vi "报警信息.vi"(11 "报警簇":T1) -> (2 "系统报警信息":string, 3 "采配水报警信息":string)   [LabVIEW 2016, in "PLC.lvlib"]
uses:
  PLC.lvlib
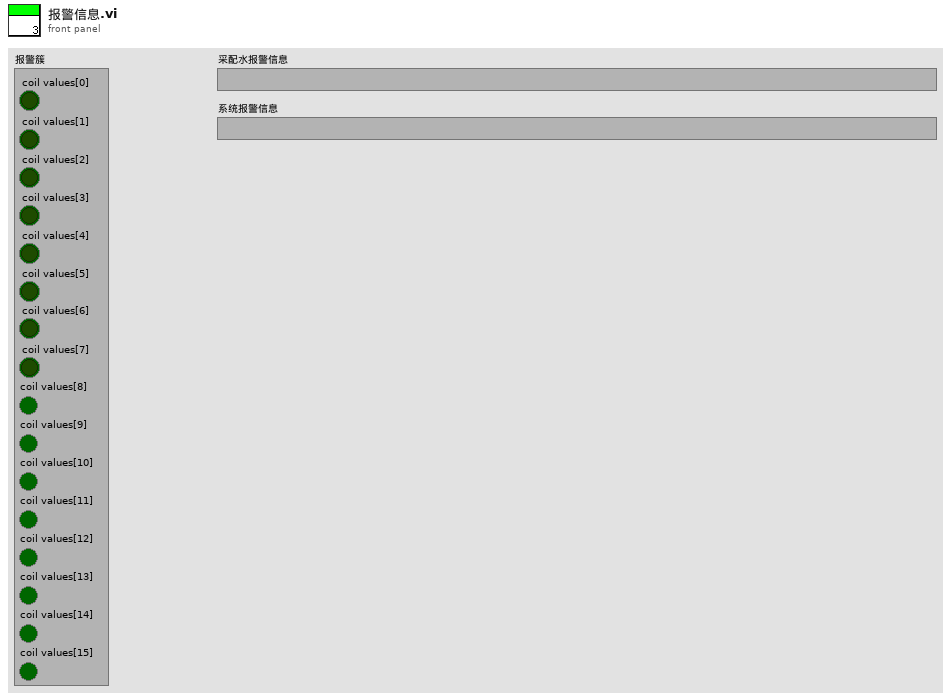
[diagram p1: front panel]
types:
  T1 = cluster{"coil values[0]":bool, "coil values[1]":bool, "coil values[2]":bool, "coil values[3]":bool, "coil values[4]":bool, "coil values[5]":bool, "coil values[6]":bool, "coil values[7]":bool, "coil values[8]":bool, "coil values[9]":bool, "coil values[10]":bool, "coil values[11]":bool, "coil values[12]":bool, "coil values[13]":bool, "coil values[14]":bool, "coil values[15]":bool}
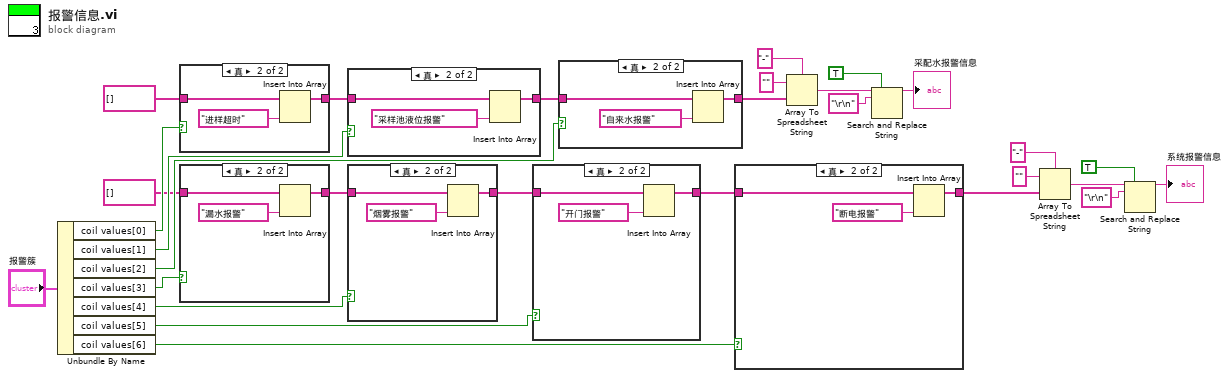
[diagram p0: block diagram]
diagram:
  n1 = Unbundle By Name("报警簇") -> ("coil values[0]"=w28:bool, "coil values[1]"=w27:bool, "coil values[2]"=w22:bool, "coil values[3]"=w21:bool, "coil values[4]"=w20:bool, "coil values[5]"=w19:bool, "coil values[6]"=w18:bool)
  n2 = case shown="真" w28 {
    tunnel: string[] [] -> [w30 w32]
    tunnel: [w30 w31] -> w23
    frame False {
    }
    frame True {
      n3 = Insert Into Array(array=w32, new element="进样超时" ("组合框")) -> (w31:string[])  [unwired: 1 in]
    }
  }
  n4 = case shown="真" w21 {
    tunnel: string[] [] -> [w34 w37]
    tunnel: [w34 w35] -> w17
    frame False {
    }
    frame True {
      n5 = Insert Into Array(array=w37, new element="漏水报警" ("组合框")) -> (w35:string[])  [unwired: 1 in]
    }
  }
  n6 = case shown="真" w27 {
    tunnel: w23 -> [w38 w41]
    tunnel: [w38 w39] -> w10
    frame False {
    }
    frame True {
      n7 = Insert Into Array(array=w41, new element="采样池液位报警" ("组合框")) -> (w39:string[])  [unwired: 1 in]
    }
  }
  n8 = case shown="真" w20 {
    tunnel: w17 -> [w42 w45]
    tunnel: [w42 w43] -> w16
    frame False {
    }
    frame True {
      n9 = Insert Into Array(array=w45, new element="烟雾报警" ("组合框")) -> (w43:string[])  [unwired: 1 in]
    }
  }
  n10 = case shown="真" w19 {
    tunnel: w16 -> [w46 w49]
    tunnel: [w46 w47] -> w15
    frame False {
    }
    frame True {
      n11 = Insert Into Array(array=w49, new element="开门报警" ("组合框")) -> (w47:string[])  [unwired: 1 in]
    }
  }
  n12 = case shown="真" w22 {
    tunnel: w10 -> [w50 w51]
    tunnel: [w50 w52] -> w9
    frame False {
    }
    frame True {
      n13 = Insert Into Array(array=w51, new element="自来水报警" ("组合框")) -> (w52:string[])  [unwired: 1 in]
    }
  }
  n14 = case shown="真" w18 {
    tunnel: w15 -> [w54 w57]
    tunnel: [w54 w55] -> w14
    frame False {
    }
    frame True {
      n15 = Insert Into Array(array=w57, new element="断电报警" ("组合框")) -> (w55:string[])  [unwired: 1 in]
    }
  }
  n16 = Array To Spreadsheet String(delimiter (Tab)="-" ("分隔符(Tab)"), array=w9, 3:"" ("格式字符串")) -> (spreadsheet string=w2:string)
  n17 = Search and Replace String(replace all?=TRUE ("替换全部？(F)"), input string=w2, search string="\r\n" ("搜索字符串")) -> (result string=→"采配水报警信息":string)  [unwired: 5 in, 3 out]
  n18 = Array To Spreadsheet String(delimiter (Tab)="-" ("分隔符(Tab)"), array=w14, 3:"" ("格式字符串")) -> (spreadsheet string=w8:string)
  n19 = Search and Replace String(replace all?=TRUE ("替换全部？(F)"), input string=w8, search string="\r\n" ("搜索字符串")) -> (result string=→"系统报警信息":string)  [unwired: 5 in, 3 out]
